vi "Table with Bemerkung und PageBreak.vi"(4 "Index":i32, 5 "Table Content":T5={"TableHeader"=[], "Table"=[], "Relative Column Widths (%)"=[], "Results"={"Results"=[], "ResultPictures"={"Yes Ctl Refnum"=refnum, "No Ctl Refnum"=refnum}, "use Pictures"=FALSE, "Image Scale (%)"=100.0, "Autoscale? (T)"=TRUE, "Horizontal Align"=3, "Position"=0}, "PositionBemerkung"=enum."before", "PageBreak"=enum."before", "TablePictures"={"Ctl Refnum In"=[], "RowOrColumn"=enum."Row", "IndexToInsert"=0, "Image Scale (%)"=[], "Autoscale? (T)"=[], "Horizontal Align"=3}, "Horizontal Align"=3} {"Horizontal Align" items=["Center", "Justified", "JustifiedAll", "Left", "Right"]; "TablePictures"."Horizontal Align" items=["Center", "Justified", "JustifiedAll", "Left", "Right"]; "Results"."Position" items=["First", "Last"]; "Results"."Horizontal Align" items=["Center", "Justified", "JustifiedAll", "Left", "Right"]}, 6 "TableFont":T1={"Font"="Arial", "Size"=10, "Colour"=0, "Bold"=FALSE, "Italic"=FALSE, "Underline"=FALSE, "Strikethrough"=FALSE, "Font Encoding"=enum."Cp1252, WinANSI"}, 7 "Bemerkungen":T3[](array[typedef]) {"Align (Left)" items=["Center", "Justified", "Justified All", "Left", "Right"]}, 8 "Fehler (Eingang, kein Fehler)":errorcluster, 11 "Context (Eingang)":refnum<class "Context.lvclass">) -> (0 "Fehler (Ausgang)":errorcluster, 3 "Context (Ausgang)":refnum<class "Context.lvclass">)   [LabVIEW 2020, in "PDF Interface.lvlib" / "PDF Interface Helper.lvlib"]
uses:
  PDF Interface Helper.lvlib
  PDFTableContentType.ctl
  PDFResults.ctl
  PDFResultPictures.ctl
  PDFCommentPosition.ctl
  PDFPageBreak.ctl
  PDFTablePictures.ctl
  PDFBemerkung.ctl
  <vilib>/Simplicity AI/SAI_PDF_API/Classes/Context/Controls/SAI_PDF_Text Align.ctl
  <vilib>/Simplicity AI/SAI_PDF_API/Classes/Context/Controls/SAI_PDF_Font.ctl
  <vilib>/Simplicity AI/SAI_PDF_API/Classes/Context/Controls/SAI_PDF_Font Encoding.ctl
  <vilib>/Simplicity AI/SAI_PDF_API/Classes/Context/Context.lvclass
panel:
  # "(Cp1252)"
  # "(Cp1252)"
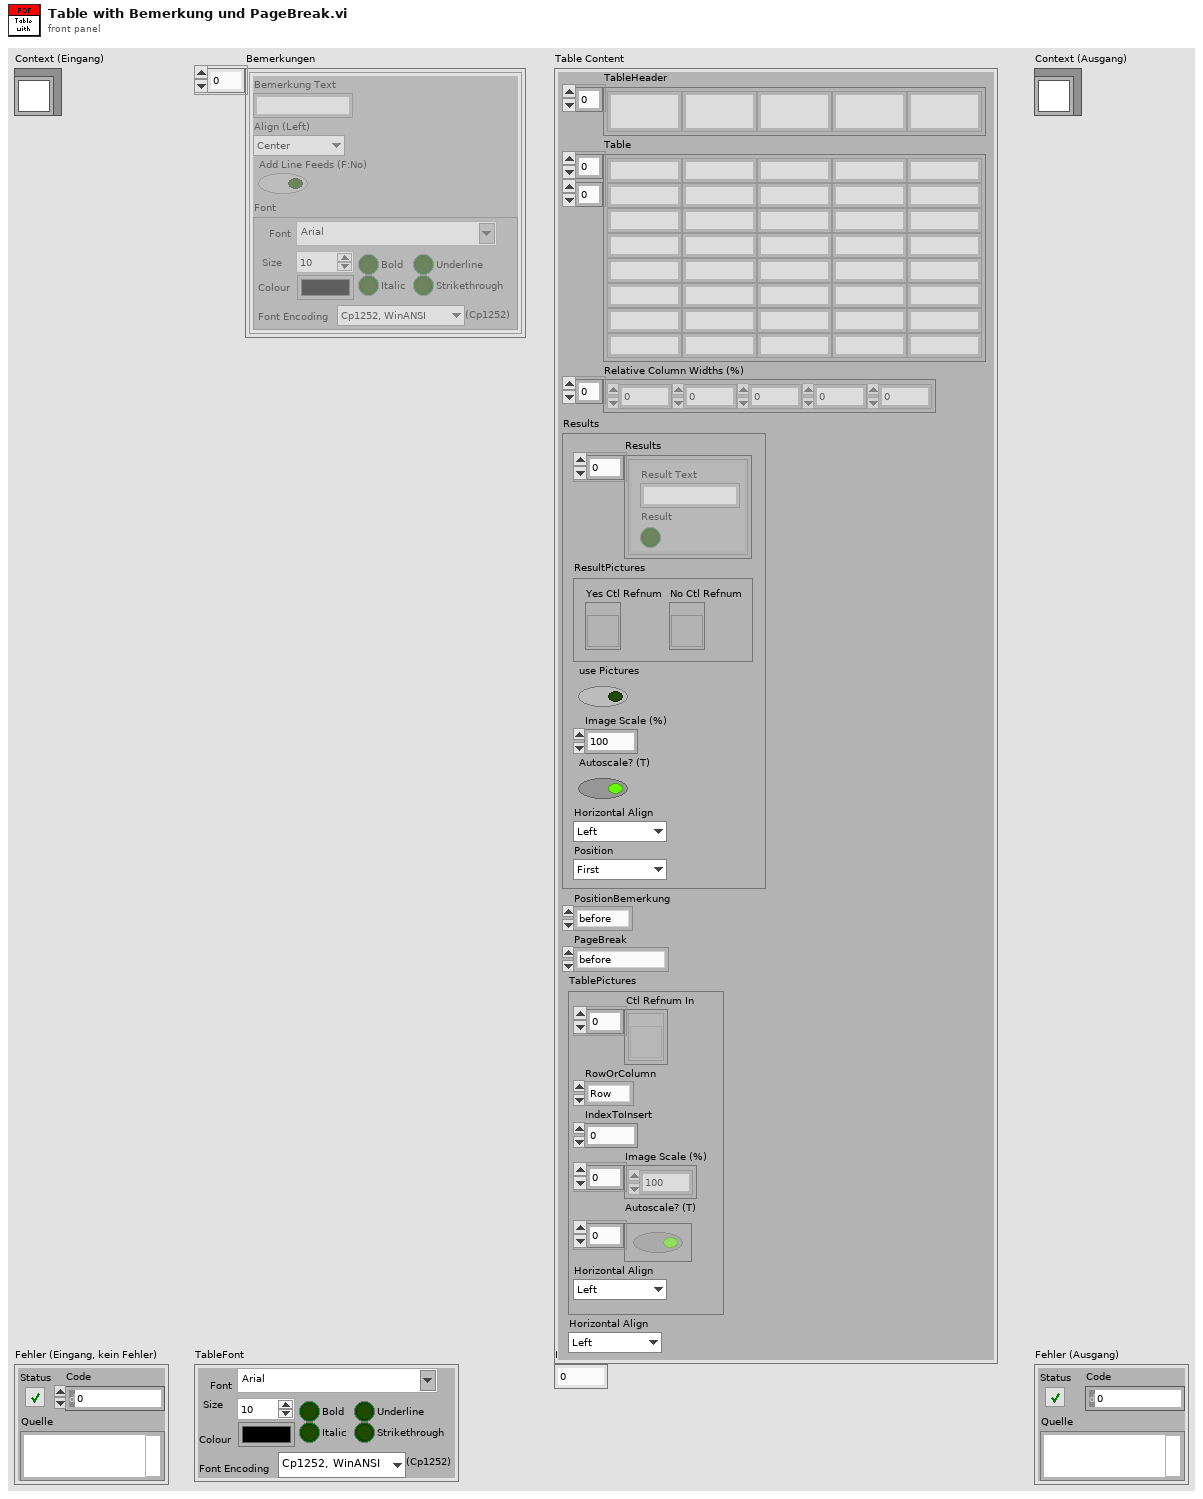
[diagram p1: front panel]
types:
  T1 = typedef "SAI_PDF_Toolkit.lvlib/Context.lvclass/SAI_PDF_Font.ctl" = cluster{"Font":string, "Size":i32, "Colour":u32, "Bold":bool, "Italic":bool, "Underline":bool, "Strikethrough":bool, "Font Encoding":T2}
  T2 = typedef "SAI_PDF_Toolkit.lvlib/Context.lvclass/SAI_PDF_Font Encoding.ctl" = enum16{"Cp1252, WinANSI", "IdentityH", "IdentityV", "Cp1250", "Cp1257", "MacRoman"}
  T3 = typedef "PDF Interface.lvlib/PDF Interface Helper.lvlib/PDFBemerkung.ctl" = cluster{"Bemerkung Text":string, "Align (Left)":T4, "Add Line Feeds (F:No)":bool, "Font":T1}
  T4 = typedef "SAI_PDF_Toolkit.lvlib/Context.lvclass/SAI_PDF_Text Align.ctl" = i32
  T5 = typedef "PDF Interface.lvlib/PDF Interface Helper.lvlib/PDFTableContentType.ctl" = cluster{"TableHeader":string[], "Table":string[][], "Relative Column Widths (%)":sgl[], "Results":T6, "PositionBemerkung":T8, "PageBreak":T9, "TablePictures":T10, "Horizontal Align":i32}
  T6 = typedef "PDF Interface.lvlib/PDF Interface Helper.lvlib/PDFResults.ctl" = cluster{"Results":cluster{"Result Text":string, "Result":bool}[], "ResultPictures":T7, "use Pictures":bool, "Image Scale (%)":sgl, "Autoscale? (T)":bool, "Horizontal Align":i32, "Position":i32}
  T7 = typedef "PDF Interface.lvlib/PDF Interface Helper.lvlib/PDFResultPictures.ctl" = cluster{"Yes Ctl Refnum":refnum<vi>, "No Ctl Refnum":refnum<vi>}
  T8 = typedef "PDF Interface.lvlib/PDF Interface Helper.lvlib/PDFCommentPosition.ctl" = enum16{"before", "after"}
  T9 = typedef "PDF Interface.lvlib/PDF Interface Helper.lvlib/PDFPageBreak.ctl" = enum16{"none", "before", "after", "after comment"}
  T10 = typedef "PDF Interface.lvlib/PDF Interface Helper.lvlib/PDFTablePictures.ctl" = cluster{"Ctl Refnum In":refnum<vi>[], "RowOrColumn":enum16{"Row", "Column"}, "IndexToInsert":u16, "Image Scale (%)":sgl[], "Autoscale? (T)":bool[], "Horizontal Align":i32}
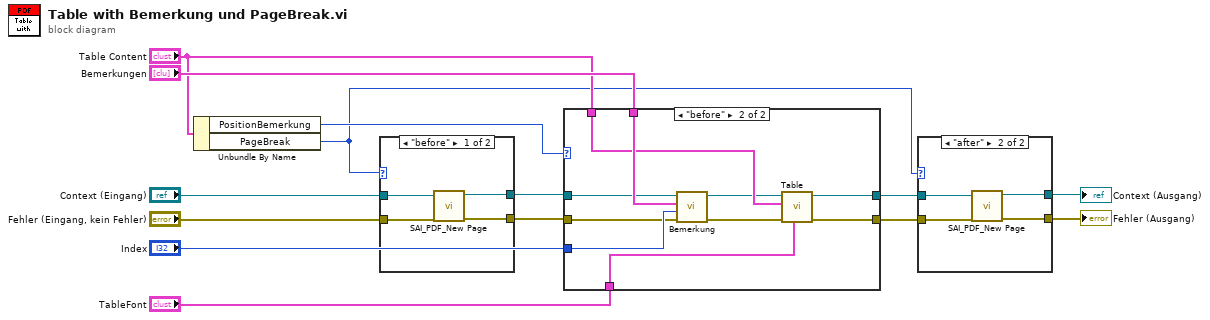
[diagram p0: block diagram]
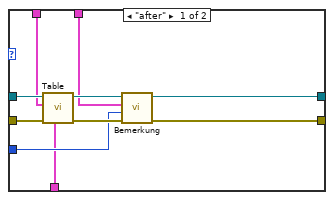
[diagram p4: hidden frame]
diagram:
  n1 = Unbundle By Name("Table Content") -> ("PositionBemerkung"=w3:T8, "PageBreak"=w2:T9)
  n2 = case shown="\"before\"" w2 {
    tunnel: "Context (Eingang)" -> [w18 w20]
    tunnel: [w17 w20] -> w6
    tunnel: "Fehler (Eingang, kein Fehler)" -> [w16 w19]
    tunnel: [w15 w19] -> w5
    frame "before" {
      n3 = call <vilib>:"SAI_PDF_New Page.vi"("error in"=w16, "Context In"=w18) -> ("error out"=w15:errorcluster, "Context Out"=w17:refnum<class "Context.lvclass">)  [unwired: 8 in]
    }
    frame "after", Default {
    }
  }
  n4 = case shown="\"before\"" w3 {
    tunnel: [w28 w37] -> w12
    tunnel: [w27 w32] -> w10
    tunnel: w6 -> [w26 w36]
    tunnel: w5 -> [w25 w35]
    tunnel: "Bemerkungen" -> [w24 w40]
    tunnel: "Table Content" -> [w23 w39]
    tunnel: "Index" -> [w22 w38]
    tunnel: "TableFont" -> [w21 w31]
    frame "after" {
      n5 = call "Table.vi"("Font"=w21, "error in"=w25, "Table Content"=w23, "Context In"=w26) -> ("error out"=w29:errorcluster, "Context Out"=w30:refnum<class "Context.lvclass">)  [unwired: 6 in]
      n6 = call "Bemerkung.vi"("Fehler (Eingang, kein Fehler)"=w29, "Index"=w22, "Bemerkung"=w24, "Context (Eingang)"=w30) -> ("Fehler (Ausgang)"=w27:errorcluster, "Context (Ausgang)"=w28:refnum<class "Context.lvclass">)  [unwired: 6 in]
    }
    frame "before" {
      n7 = call "Bemerkung.vi"("Fehler (Eingang, kein Fehler)"=w35, "Index"=w38, "Bemerkung"=w40, "Context (Eingang)"=w36) -> ("Fehler (Ausgang)"=w34:errorcluster, "Context (Ausgang)"=w33:refnum<class "Context.lvclass">)  [unwired: 6 in]
      n8 = call "Table.vi"("Font"=w31, "error in"=w34, "Table Content"=w39, "Context In"=w33) -> ("error out"=w32:errorcluster, "Context Out"=w37:refnum<class "Context.lvclass">)  [unwired: 6 in]
    }
  }
  n9 = case shown="\"after\"" w2 {
    tunnel: w12 -> [w42 w46]
    tunnel: [w42 w45] -> w11
    tunnel: w10 -> [w41 w44]
    tunnel: [w41 w43] -> w9
    frame "before", Default {
    }
    frame "after" {
      n10 = call <vilib>:"SAI_PDF_New Page.vi"("error in"=w44, "Context In"=w46) -> ("error out"=w43:errorcluster, "Context Out"=w45:refnum<class "Context.lvclass">)  [unwired: 8 in]
    }
  }
  "Fehler (Ausgang)" <- w9
  "Context (Ausgang)" <- w11
